vi "niDTS BT INSTR TX Configure OBW.vi"(8 "error in (no error)":errorcluster, 11 "niDTS BT INSTR TX in":refnum<class "niDTS BT INSTR TX.lvclass">) -> (0 "error out":errorcluster, 3 "niDTS BT INSTR TX out":refnum<class "niDTS BT INSTR TX.lvclass">)   [LabVIEW 2015, in "niDTS BT.lvlib" / "niDTS BT INSTR TX.lvclass"]
doc: "Sets:\n\n* TriggerThreshold\n* Trigger Source\n* MinQuietTimeDuration\n* TriggerTimeout"
uses:
  niDTS BT INSTR TX.lvclass
  niDTS BT INSTR TX.lvclass/niDTS BT INSTR TX.ctl
  RiviInstDriver/niRfsaBT/Objects/niRfsaBt.lvclass
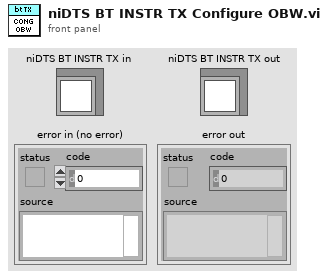
[diagram p1: front panel]
types:
  T1 = typedef "niRfsaBT.lvclass/niRfsaBT INC Handle.ctl" = refnum<data-value>
  T2 = enum16{"RMS", "LOG", "SCALAR", "MAX", "MIN", "VECTOR"}
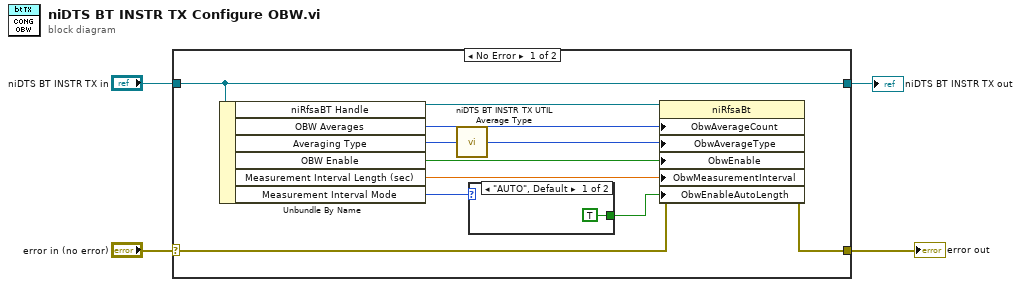
[diagram p0: block diagram]
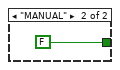
[diagram p2: hidden frame]
diagram:
  n1 = case shown="No Error" "error in (no error)" {
    selector: "error in (no error)" -> [w15 w19]
    tunnel: [w14 w19] -> w3
    tunnel: "niDTS BT INSTR TX in" -> [w12 w18]
    tunnel: [w12 w18] -> w1
    frame No Error {
      n2 = Unbundle By Name(w12) -> ("niRfsaBT Handle"=w13:T1, "OBW Averages"=w10:i32, "Averaging Type"=w9:T2, "OBW Enable"=w8:bool, "Measurement Interval Length (sec)"=w11:dbl, "Measurement Interval Mode"=w6:enum16{"AUTO", "MANUAL"})
      n3 = call "niDTS BT INSTR TX UTIL Average Type.vi"("Type In"=w9) -> ("Type Out"=w7:enum16{"RMS", "LOG", "SCALar", "MAX", "MIN"})  [unwired: 14 in]
      n4 = case shown="\"AUTO\", Default" w6 {
        tunnel: [TRUE ("CONFigure:RFSA:BLUetooth:MEASurement:OBW:INTerval:LENGth:AUTO:ObwEnableAutoLength") FALSE ("CONFigure:RFSA:BLUetooth:MEASurement:OBW:INTerval:LENGth:AUTO:ObwEnableAutoLength")] -> w5
        frame "AUTO", Default {
        }
        frame "MANUAL" {
        }
      }
      n5 = property class="niRfsaBt"(reference=w13, error in=w15, "ObwAverageCount"=w10, "ObwAverageType"=w7, "ObwEnable"=w8, "ObwMeasurementInterval"=w11, "ObwEnableAutoLength"=w5) -> (error out=w14:errorcluster)  [unwired: 1 out]
    }
    frame Error {
    }
  }
  "error out" <- w3
  "niDTS BT INSTR TX out" <- w1
